vi "QE Read.vi"   [LabVIEW 2013, in "LVH-LINX.lvlib"]
doc: "Read the counter value(s) of the specifed quadrature encoder channel(s)."
uses:
  LVH-LINX.lvlib
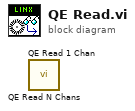
[diagram p0: block diagram]
diagram:
  n1 = call "QE Read N Chans.vi"() -> ()  [unwired: 9 in, 3 out]
  n2 = call "QE Read 1 Chan.vi"() -> ()  [unwired: 9 in, 3 out]
